vi "Method Flying with wings.vi"(0 "Flying Behaviors in":refnum<class "Flying Behaviors.lvclass">, 11 "error in (no error)":errorcluster) -> (4 "Flying Behaviors out":refnum<class "Flying Behaviors.lvclass">, 15 "error out":errorcluster)   [LabVIEW 2021, in "Flying Behaviors.lvclass"]
uses:
  Flying Behaviors.lvclass
panel:
  # "Connector Pane"
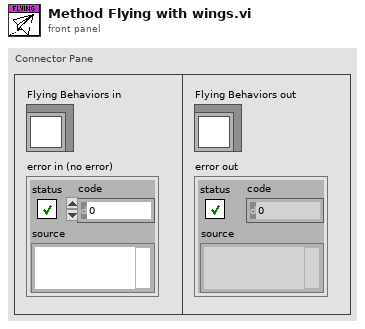
[diagram p1: front panel]
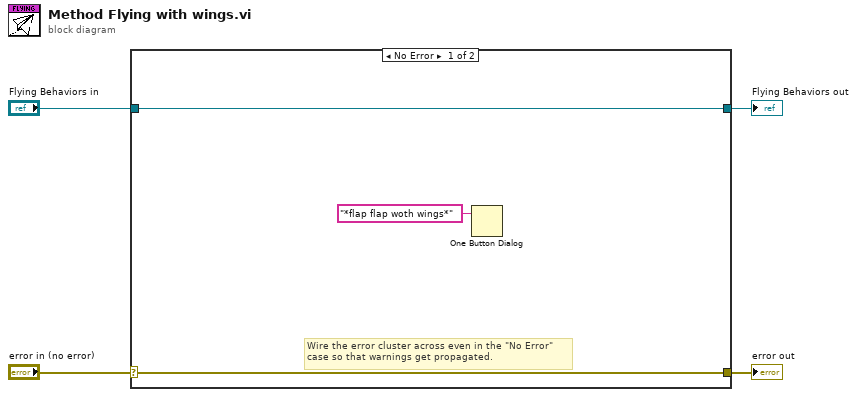
[diagram p0: block diagram]
diagram:
  n1 = case shown="No Error" "error in (no error)" {
    selector: "error in (no error)" -> [w6 w9]
    tunnel: [w6 w9] -> w3
    tunnel: [w7 w8] -> w1
    tunnel: "Flying Behaviors in" -> [w7 w8]
    frame No Error {
      # "Wire the error cluster across even in the \"No Error\"\ncase so that warnings get propagated."
      n2 = One Button Dialog(message="*flap flap woth wings*") -> ()  [unwired: 1 in, 1 out]
    }
    frame Error {
    }
  }
  "error out" <- w3
  "Flying Behaviors out" <- w1
